vi "Set Speed and Acceleration.vi"(4 "Units (0: data)":u16(ring) items=["device units", "microns/s, microns/s^2", "mm/s, mm/s^2", "inches/s, inches/s^2", "degrees/s, degrees/s^2"], 5 "New Acceleration (0)":dbl, 7 "New Speed (0)":dbl, 8 "error in (no error)":errorcluster, 9 "Device and Axis":string, 10 "Microstep Size (0)":dbl, 11 "VISA resource name":refnum<visa-resource-name>) -> (0 "error out":errorcluster, 3 "VISA resource name out":refnum<visa-resource-name>)   [LabVIEW 2018, in "Zaber A Series.lvlib"]
doc: "Sets the speed and/or acceleration of a device to a new value. The desired speed and accel are inputs. If either is not connected or the value is 0, then it won't be updated. The units for the speed and acceleration can be selected with the Units input. 'Data' units are the default, and other unit selections require the Microstep Size for the device to be input. If you'd like to specify a Device and Axis to adjust the settings of, specify this input.\n\nThis VI requires that the Initialize VI has been called with the same serial port."
uses:
  Zaber A Series.lvlib
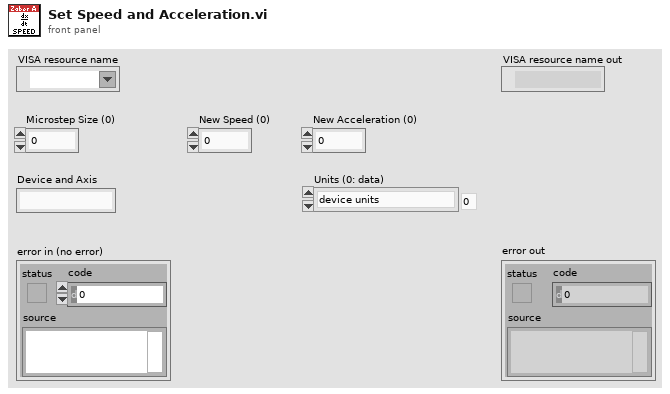
[diagram p1: front panel]
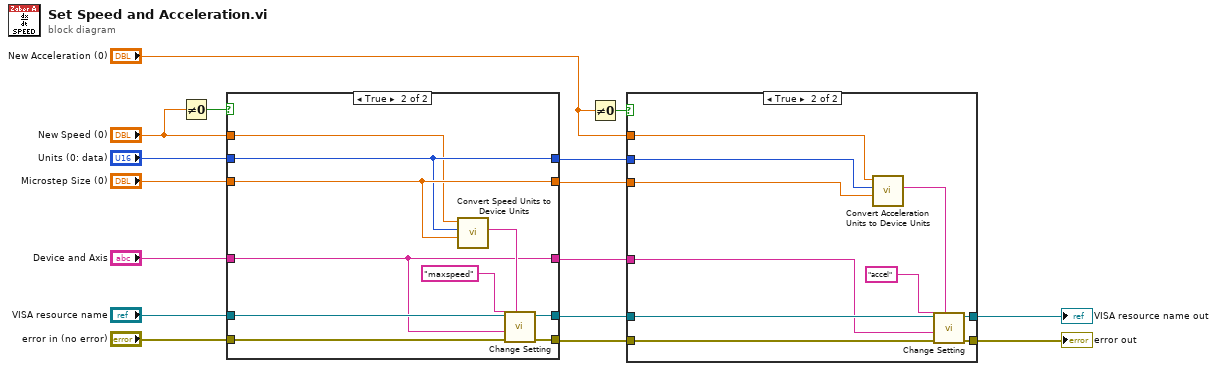
[diagram p0: block diagram]
diagram:
  n1 = Not Equal To 0?(x="New Speed (0)") -> (x != 0?=w11:bool)
  n2 = case shown="True" w11 {
    tunnel: "VISA resource name" -> [w21 w29]
    tunnel: "error in (no error)" -> [w20 w30]
    tunnel: "New Speed (0)" -> [_ w22]
    tunnel: "Microstep Size (0)" -> [w18 w24]
    tunnel: "Units (0: data)" -> [w19 w23]
    tunnel: [w21 w28] -> w14
    tunnel: [w20 w27] -> w13
    tunnel: "Device and Axis" -> [w17 w25]
    tunnel: [w17 w25] -> w7
    tunnel: [w18 w24] -> w5
    tunnel: [w19 w23] -> w4
    frame False {
    }
    frame True {
      n3 = call "Convert Speed Units to Device Units.vi"("Microstep Size (0)"=w24, "Units (0: device speed units)"=w23, "Speed (0)"=w22) -> ("Device Speed (String)"=w26:string)  [unwired: 6 in, 2 out]
      n4 = call "Change Setting.vi"("Data"=w26, "error in (no error)"=w30, "Device and Axis"=w25, "Setting"="maxspeed" ("Common Settings"), "VISA resource name"=w29) -> ("error out"=w27:errorcluster, "VISA resource name out"=w28:refnum<visa-resource-name>)  [unwired: 5 in]
    }
  }
  n5 = Not Equal To 0?(x="New Acceleration (0)") -> (x != 0?=w10:bool)
  n6 = case shown="True" w10 {
    tunnel: w14 -> [w33 w39]
    tunnel: [w33 w43] -> w2
    tunnel: w13 -> [w32 w41]
    tunnel: [w32 w42] -> w1
    tunnel: w5 -> [_ w34]
    tunnel: w4 -> [_ w35]
    tunnel: w7 -> [_ w38]
    tunnel: "New Acceleration (0)" -> [_ w36]
    frame False {
    }
    frame True {
      n7 = call "Convert Acceleration Units to Device Units.vi"("Microstep Size (0)"=w34, "Units (0: device acceleration units)"=w35, "Acceleration (0)"=w36) -> ("Device Acceleration (String)"=w37:string)  [unwired: 6 in, 2 out]
      n8 = call "Change Setting.vi"("Data"=w37, "error in (no error)"=w41, "Device and Axis"=w38, "Setting"="accel" ("Common Settings"), "VISA resource name"=w39) -> ("error out"=w42:errorcluster, "VISA resource name out"=w43:refnum<visa-resource-name>)  [unwired: 5 in]
    }
  }
  "VISA resource name out" <- w2
  "error out" <- w1
